vi "Update ZStep to AOL params.vi"(8 "error in (no error)":errorcluster) -> (0 "error out":errorcluster)   [LabVIEW 2020]
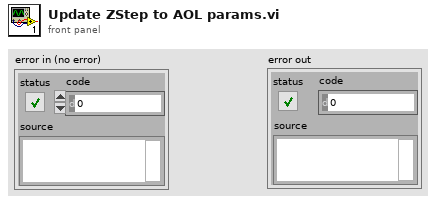
[diagram p1: front panel]
types:
  T1 = typedef "Reference_Globals.ctl" = cluster{"Refrence data path":path, "Reference Rectangle":i16[][], "AOL Z":dbl, "No of pixels in a miniscan ":i32[], "Threshold":i16[], "No of miniscans":i32[], "Full Frame Size":u16, "Reference Image":T2, "dwelltime":dbl, "Zoom":dbl, "Field of View":dbl, "Z Step":i8, "Z pixels":i32, "Z Lines":u8, "Z Ignore":u8, "Laser":u8}
  T2 = typedef "IMAQ Image.ctl" = refnum<image>
  T3 = typedef "AOL_Globals.ctl" = cluster{"Imaging Protocol":T4, "Number of POI":u16, "Number of Miniscans":u16, "Number of Trials":u16, "Number of Cycles ":u64, "# Averaged Frames":u16, "Laser power (%)":u8, "Pockels (V)":dbl, "Acquisition Length (sec)":dbl, "Fill time (us)":dbl, "POI Dwell time (us)":dbl, "Miniscan Dwell time per pixel (us)":dbl, "PMT 1":dbl, "PMT 2":dbl, "Back Apperture (mA)":dbl, "Frame Size":T5, "Center Frequency":dbl, "Field of View (norm)":dbl, "DwellTime (us)":dbl, "Wavelength (nm)":dbl, "Zoom":dbl, "AOL Z":dbl, "AOL Mode":T6, "GridXY":dbl, "GridZ":dbl, "TriggerPeriod (sec)":dbl, "Number of Pixels in Miniscan":u16, "Experiment folder path":path, "X centre":dbl, "Y centre":dbl, "Angle (degrees)":dbl, "Plane Mode":T7, "Threshold":u16[], "Regenerate Chirps":bool, "Rectangle ROI length (pixels)":u16, "Rectangle ROI height (pixels)":u16, "AOD fill":u16, "StartupDelay":i32, "Samples Wait after Trigger":u16, "Slip Cycle":u32, "Add Cycle":bool, "Functional Mode":T8, "Z Start":dbl, "Z Stop":dbl, "# Planes":i32, "Total Pixels":i32, "Variable Miniscan Pixels":u16[], "Use Variable Length":bool, "Use Variable Resolution":bool, "Laser power (%) at Z Start":u8, "Laser power (%) at Z Stop":u8, "Ref Z Step":i8, "Ref Dwell Time (us)":dbl, "Field of View (um)":dbl}
  T4 = typedef "Imaging Protocols enum.ctl" = enum16{"AOL Z-Stack", "Motor Z Stack", "Functional Acquisition", "Single Plane Acquisition", "Volume Acquisition", "Live Imaging", "Live Plane Imaging", "Live Volume Imaging"}
  T5 = typedef "Frame Size.ctl" = u16
  T6 = typedef "AOL modes.ctl" = enum16{"Raster", "Structural", "Pointing", "Mini Scan", "Alignment"}
  T7 = typedef "Plane Mode.ctl" = u16
  T8 = typedef "Functional Mode.ctl" = enum16{"Point", "Line", "Patch", "Plane", "Volume"}
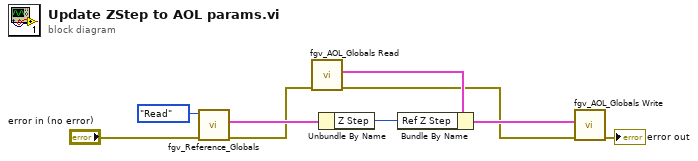
[diagram p0: block diagram]
diagram:
  n1 = call "fgv_Reference_Globals.vi"("error in (no error)"="error in (no error)", "Function"=enum16{"Intialize", "Write", "Read", "Clear"}."Read") -> ("error out"=w2:errorcluster, "Reference Data"=w8:T1)  [unwired: 8 in]
  n2 = call "fgv_AOL_Globals Read.vi"("error in (no error)"=w2) -> ("error out"=w5:errorcluster, "AOL_Globals"=w7:T3)  [unwired: 8 in, 1 out]
  n3 = Unbundle By Name(w8) -> ("Z Step"=w3:i8)
  n4 = Bundle By Name(cluster=w7, "Ref Z Step"=w3) -> (w6:T3)
  n5 = call "fgv_AOL_Globals Write.vi"("error in (no error)"=w5, "AOL_Globals"=w6) -> ("error out"=→"error out":errorcluster)  [unwired: 9 in]
